vi "myRIO_BRig_RT__Case_Exp_State_Wrong.vi"(10 "input_state":T1, 11 "input_dataCurrent":u16[](array[numeric])) -> (2 "output_state":T1, 3 "output_dataCurrent":u16[](array[numeric]))   [LabVIEW 2014]
uses:
  myRIO_BRig_RT__Case_Exp_stateList.ctl
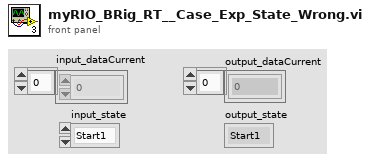
[diagram p1: front panel]
types:
  T1 = typedef "myRIO_BRig_RT__Case_Exp_stateList.ctl" = enum16{"Start1", "Start2", "Start3", "saveSettings1", "saveSettings2", "saveSettings3", "saveSettings4", "saveSettings_LC_ENL_l1", "saveSettings_LC_ENL_l2", "saveSettings_LC_Cue_l1", "saveSettings_LC_Cue_l2", "saveSettings6_LC_l1_Other", "SaveSettings6_LC_l2_Other", "setSettings_Audio", "setSettings_Laser", "initBlock_pre", "initBlock", "initBlock2", "initBlock_post", "initTrial_pre", "initTrial", "initTrial2", "initTrial3", "initTrial4", "initTrial_LC_ENL1", "initTrial_LC_Cue1", "initTrial_LC_Cue1_2", "initTrial_LC_Sel", "initTrial_post", "ENL1_pre", "ENL1", "ENL1_post", "ENL1Penalty_pre", "ENL1Penalty", "ENL2_pre", "ENL2", "ENL2Penalty_pre", "ENL2Penalty", "Cue1_pre", "Cue1", "Cue1_post", "Cue1Penalty_pre", "Cue1Penalty", "Cue2_pre", "Cue2", "Cue2Penalty_pre", "Cue2Penalty", "Selection_pre", "Selection", "Select_post", "SelectReward_pre", "SelectReward", "SelectRewardPost_pre", "SelectRewardPost", "SelectWrong_pre", "SelectWrong", "SelectWrong_post", "SelectTimeout_pre", "SelectTimeout", "SelectTimeout_post", "endTrial_pre", "endTrial1", "endTrial2", "endTrial3", "endTrial_post", "endBlock_pre", "endBlock", "endBlock_post", "endExp", "commConnect", "commUpload_pre", "commUpload_dataBlock", "commUpload_dataCurrent", "commUpload_dataExp", "commUpload_dataLC", "commUpload_dataTrial", "commUpload_post", "saveData_pre", "saveData_dataBlock", "saveData_dataCurrent", "saveData_dataExp", "saveData_dataLC", "saveData_dataTrial", "saveData_post", "empty_endBlock1", "empty_endBlock2", "empty_endTrial1", "empty_endTrial2", "empty_endTrial3", "empty_endTrial4", "empty_endTrial5", "dummyState", "dummyState_endBlock"}
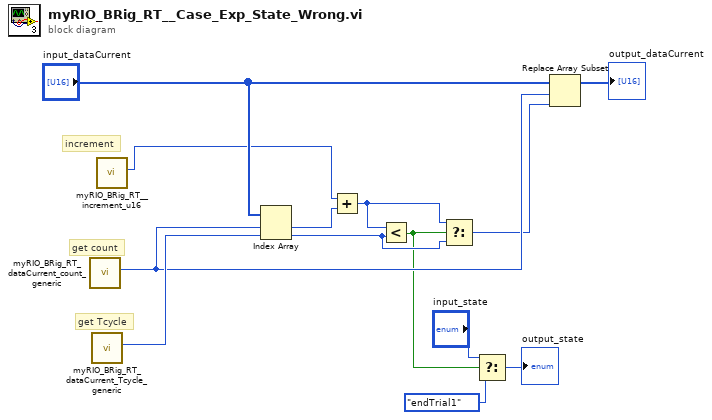
[diagram p0: block diagram]
diagram:
  # "increment"
  # "get Tcycle"
  # "get count"
  n1 = call "myRIO_BRig_RT_dataCurrent_count_generic.vi"() -> ("output_count_generic"=w9:i32)  [unwired: 11 in]
  n2 = call "myRIO_BRig_RT_dataCurrent_Tcycle_generic.vi"() -> ("output_Tcycle_generic"=w11:i32)  [unwired: 11 in]
  n3 = call "myRIO_BRig_RT__increment_u16.vi"() -> ("output_increment__u16"=w5:u16)  [unwired: 11 in]
  n4 = Index Array(array="input_dataCurrent", index #1=w9, index #2=w11) -> (element #1=w10:u16, element #2=w8:u16)
  n5 = Add(x=w5, y=w10) -> (x+y=w4:u16)
  n6 = Less?(x=w4, y=w8) -> (x < y?=w6:bool)
  n7 = Select(t=w4, s=w6, f=w8) -> (s? t:f=w7:u16)
  n8 = Select(t="input_state", s=w6, f=myRIO_BRig_RT__Case_Exp_stateList."endTrial1" ("Enum")) -> (s? t:f=→"output_state":T1)
  n9 = Replace Array Subset(array="input_dataCurrent", new element=w7, index=w9) -> (→"output_dataCurrent":u16[])
